vi "通过静态VI引用调用VI.vi"() -> ()   [LabVIEW 2013]
uses:
  <vilib>/Platform/TimedLoop/XDataNode/timing_clust.ctl
  <vilib>/Platform/TimedLoop/XDataNode/nitl_modes.ctl
  <vilib>/Platform/TimedLoop/XDataNode/wakeup.ctl
  <vilib>/Platform/TimedLoop/XDataNode/XDataNode.xnode
  <vilib>/Platform/TimedLoop/XDataNode/XDNodeRunTimeDep.lvlib
panel:
  out "应用程序:所有内存中的VI":string[](array[string])
  out "result":dbl
  in  "y":dbl
  in  "x":dbl
  in  "停止":bool
  in  "VI":i32(listbox)
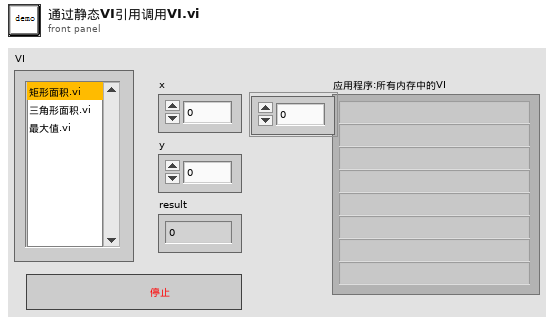
[diagram p1: front panel]
types:
  T1 = typedef "XDNodeRunTimeDep.lvlib/timing_clust.ctl" = cluster{"Expected End [f-1]":u64, "Actual End [f-1]":u64, "Finished Late? [f-1]":bool, "Expected End [i-1]":u64, "Actual End [i-1]":u64, "Finished Late? [i-1]":bool, "Expected Start [i]":u64, "Actual Start [i]":u64, "Expected Start [f]":u64, "Actual Start [f]":u64, "Source Name":string, "Structure Name":string, "Period":i64, "Deadline":i64, "Offset":i64, "Start":i64, "Priority":i32, "Timeout":i32, "Mode":T2, "Wakeup Reason":T3, "Error":errorcluster, "Source Type":string, "Secondary Source Type":string, "Global End Time":u64, "Global Start Time":u64, "Frame Duration":u64, "Iteration Duration":u64, "Assigned CPU":i32, "I/O Scan Engine Mode":u32}
  T2 = typedef "XDNodeRunTimeDep.lvlib/nitl_modes.ctl" = enum32{"No Change", "Process missed periods, maintain original phase", "Discard missed periods, maintain original phase", "Process missed periods, ignore original phase", "Discard missed periods, ignore original phase"}
  T3 = typedef "XDNodeRunTimeDep.lvlib/wakeup.ctl" = enum32{"Normal", "Aborted", "Asynchronous wakeup", "Timing source error", "Timed loop error", "Timeout"}
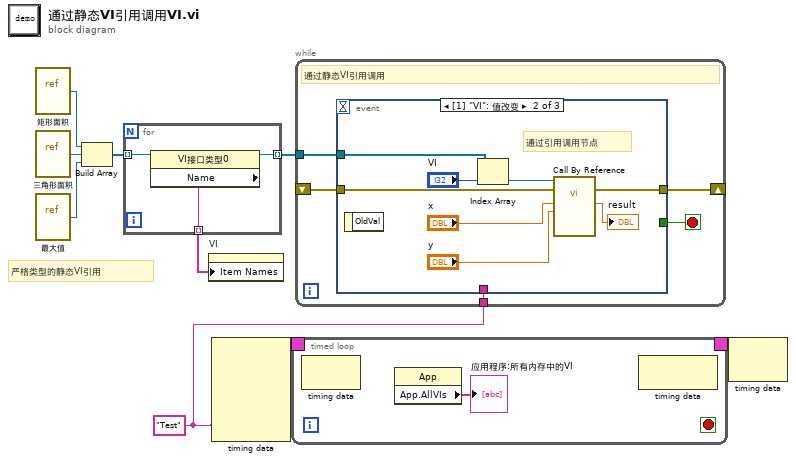
[diagram p0: block diagram]
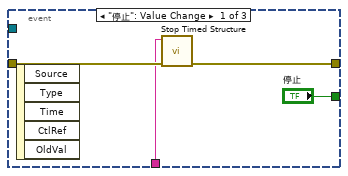
[diagram p2: hidden frame]
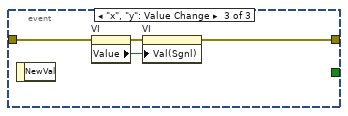
[diagram p3: hidden frame]
diagram:
  w1 = "Test" ("结构名称")
  # "严格类型的静态VI引用"
  n1 = vi-ref "矩形面积.vi"() -> (w9:refnum<vi>)
  n2 = vi-ref "三角形面积.vi"() -> (w8:refnum<vi>)
  n3 = vi-ref "最大值.vi"() -> (w7:refnum<vi>)
  n4 = Build Array(w9, w8, w7) -> (w6:refnum<vi>[])
  n5 = for {
    tunnel: w6 -> [w12] mode=indexing
    tunnel: [w11] -> w5 mode=indexing
    tunnel: [w10] -> w4 mode=indexing
    n6 = property class="VI接口类型0"(reference=w12) -> (reference out=w10:refnum<vi>, "Name"=w11:string)  [unwired: 1 in, 1 out]
  }
  n7 = property on="VI" class="LstBox (严格)"("Item Names"=w5) -> ()  [unwired: 2 in, 2 out]
  n8 = node-c288(w1) -> (w3:T1)  [unwired: 4 in]
  n9 = timed-loop {
    timing: w3 -> [_]
    timing-out: [_] -> w2
    stop <- _ stop-if-true
    n10 = node-c288() -> ()  [unwired: 1 in, 1 out]
    n11 = property class="App"() -> ("App.AllVIs"=→"应用程序:所有内存中的VI":string[])  [unwired: 2 in, 2 out]
    n12 = node-c288() -> ()  [unwired: 1 in, 1 out]
  }
  n13 = while {
    shift-right: [w17] -> _
    shift-left: _ -> [w18]
    tunnel: w4 -> [w19]
    tunnel: w1 -> [w16]
    stop <- w20 stop-if-true
    # "通过静态VI引用调用"
    n14 = event shown="[1] \"VI\": 值改变" {
      selector: _ -> [_ _ _]
      dyn-events: _ -> [_ _ _]
      timeout: _ -> [_ _ _]
      tunnel: ["停止" _ _] -> w20
      tunnel: w19 -> [_ w32 _]
      tunnel: w18 -> [w23 w26 w34]
      tunnel: [w22 w25 w33] -> w17
      tunnel: w16 -> [w21 _ _]
      event "停止": Value Change {
        n15 = event-data() -> ()  [unwired: 1 in, 5 out]
        n16 = call <vilib>:"Stop Timed Structure.vi"("error in (no error)"=w23, "name"=w21) -> ("error out"=w22:errorcluster)  [unwired: 9 in]
      }
      event "VI": Value Change {
        # "通过引用调用节点"
        n17 = event-data() -> ()  [unwired: 1 in, 1 out]
        n18 = Index Array(array=w32, index="VI") -> (element=w27:refnum<vi>)
        n19 = call-by-ref "?"(reference=w27, error in=w26, "y"="y", "x"="x") -> (error out=w25:errorcluster, "result"=→"result":dbl)  [unwired: 9 in, 1 out]
      }
      event "x", "y": Value Change {
        n20 = event-data() -> ()  [unwired: 1 in, 1 out]
        n21 = property on="VI" class="LstBox (严格)"(error in=w34) -> (error out=w36:errorcluster, "Value"=w35:i32)  [unwired: 1 in, 1 out]
        n22 = property on="VI" class="LstBox (严格)"(error in=w36, "Val(Sgnl)"=w35) -> (error out=w33:errorcluster)  [unwired: 1 in, 1 out]
      }
    }
  }
  n23 = node-c288(w2) -> ()  [unwired: 1 out]
